vi "svl_Log View for Peak Level (N Ch) (single value).vi"(7 "scaled signals [EU]":waveform(dbl)[](array[waveform]), 8 "error in (no error)":errorcluster, 10 "dB On (T)":bool=TRUE, 11 "peak levels [EU]":dbl[](array[numeric]) format="%.2f") -> (0 "error out":errorcluster, 2 "unit label [ ]":string[](array[string]), 3 "peak levels [EU]":dbl[](array[numeric]) format="%.2f")   [LabVIEW 2017]
uses:
  <vilib>/addons/_NISVFA/_Shared subVIs/Common/svc_Engineering Units to Unit Label.vi
  <vilib>/addons/_NISVFA/_Shared subVIs/Common/svc_Unit Label to Engineering Units.vi
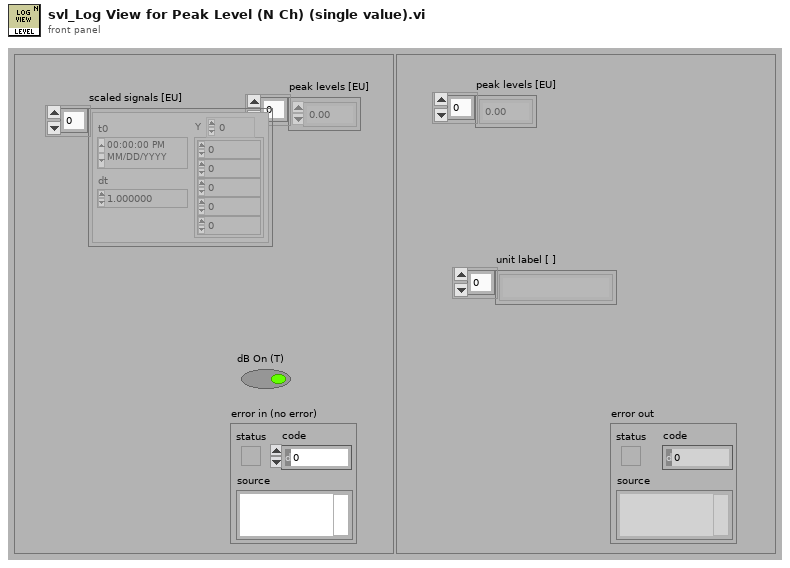
[diagram p1: front panel]
types:
  T1 = typedef "svc_Channel Info.ctl" = cluster{"sensor sensitivity":dbl, "engineering units":T2, "dB reference":dbl, "custom label":string, "weighting filter":T3, "pregain":dbl}
  T2 = typedef "svc_Engineering Units Text Ring.ctl" = u16
  T3 = typedef "svc_Weighting Filter Text Ring.ctl" = u16
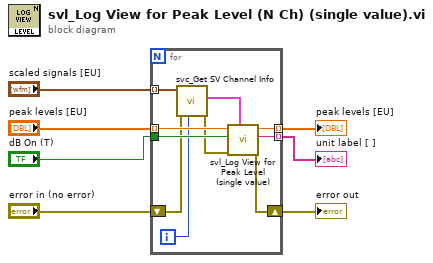
[diagram p0: block diagram]
diagram:
  n1 = for {
    tunnel: "peak levels [EU]" -> [w16] mode=indexing
    tunnel: "dB On (T)" -> [w14]
    tunnel: "scaled signals [EU]" -> [w12] mode=indexing
    tunnel: [w15] -> w5 mode=indexing
    tunnel: [w13] -> w4 mode=indexing
    shift-right: [w17] -> w1
    shift-left: "error in (no error)" -> [w11]
    i -> [w8]
    n2 = call <vilib>:"svc_Get SV Channel Info.vi"("channel index"=w8, "error in (no error)"=w11, "scaled signal [EU]"=w12) -> ("error out"=w10:errorcluster, "channel info"=w9:T1)  [unwired: 3 in, 4 out]
    n3 = call <vilib>:"svl_Log View for Peak Level (single value).vi"("channel info"=w9, "error in (no error)"=w10, "dB On (T)"=w14, "peak level [EU]"=w16) -> ("error out"=w17:errorcluster, "unit label"=w13:string, "peak level [EU]"=w15:dbl)  [unwired: 5 in]
  }
  "unit label [ ]" <- w4
  "peak levels [EU]" <- w5
  "error out" <- w1
